vi "locker-Create.vi"(8 "error in (no error)":errorcluster) -> (0 "error out":errorcluster, 3 "locker out":refnum<queue>)   [LabVIEW 2017]
doc: "Creates a locker, a queue-based mutual exclusion object, and returns its reference. The queue is seeded with one element so the first locker-lock call can take it."
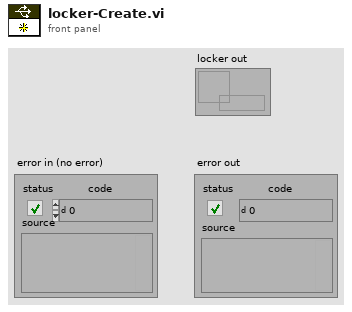
[diagram p1: front panel]
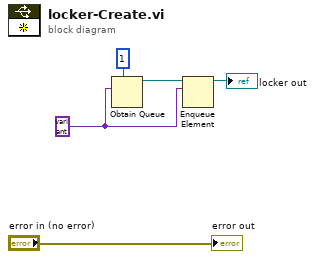
[diagram p0: block diagram]
diagram:
  w2 = variant
  n1 = Obtain Queue(max queue size (-1, unlimited)=1, element data type=w2) -> (queue out=w3:refnum<queue>)  [unwired: 3 in, 2 out]
  n2 = Enqueue Element(queue=w3, element=w2) -> (queue out=→"locker out":refnum<queue>)  [unwired: 2 in, 2 out]
  "error out" <- "error in (no error)"
